vi "Create Indicator.vi"(0 "result cluster":refnum<vi>, 5 "vi reference":refnum<vi>, 7 "ctl refnum":refnum<vi>, 11 "error in":errorcluster) -> (15 "error out":errorcluster)   [LabVIEW 2021, in "Converter.lvlib"]
uses:
  Converter.lvlib
  <vilib>/Utility/miscctls.llb/LVPositionTypeDef.ctl
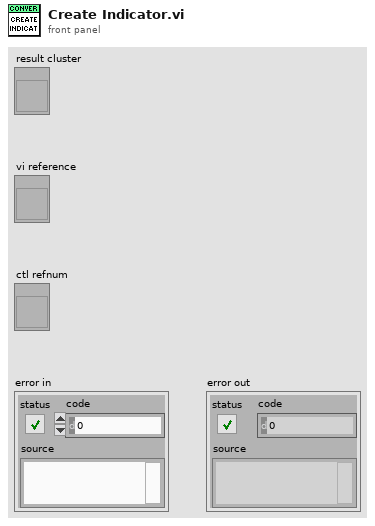
[diagram p1: front panel]
types:
  T1 = typedef "LVPositionTypeDef.ctl" = cluster{"Left":i32, "Top":i32}
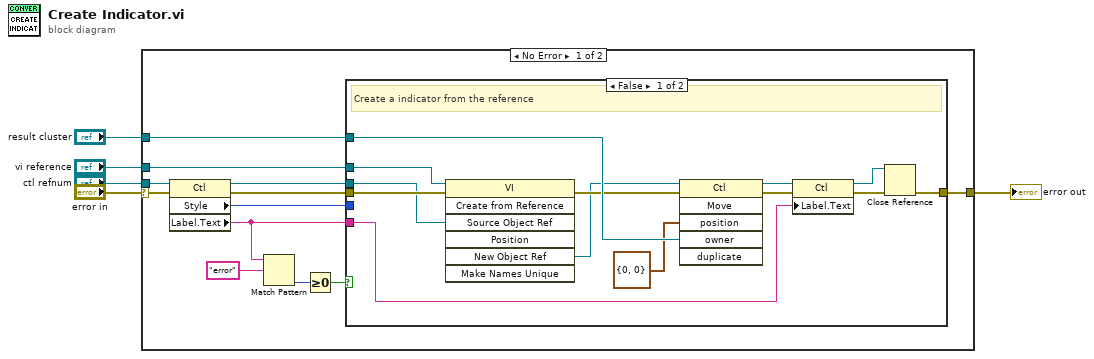
[diagram p0: block diagram]
diagram:
  n1 = case shown="No Error" "error in" {
    selector: "error in" -> [w17 w32]
    tunnel: "ctl refnum" -> [w16 _]
    tunnel: "vi reference" -> [w14 _]
    tunnel: [w10 w32] -> w2
    tunnel: "result cluster" -> [w8 _]
    frame No Error {
      n2 = property class="Ctl"(reference=w16, error in=w17) -> (reference out=w15:refnum<vi>, error out=w9:errorcluster, "Style"=w7:u32, "Label.Text"=w11:string)
      n3 = Match Pattern(string=w11, regular expression="error") -> (offset past match=w6:i32)  [unwired: 1 in, 3 out]
      n4 = Greater Or Equal To 0?(x=w6) -> (x >= 0?=w13:bool)
      n5 = case shown="False" w13 {
        tunnel: w7 -> [_ _]
        tunnel: w8 -> [w27 _]
        tunnel: w9 -> [w30 w31]
        tunnel: w15 -> [w26 _]
        tunnel: [w29 w31] -> w10
        tunnel: w11 -> [w28 _]
        tunnel: w14 -> [w25 _]
        frame False {
          # "Create a indicator from the reference"
          n6 = invoke class="VI" method="Create from Reference"(reference=w25, error in=w30, "Source Object Ref"=w26) -> (error out=w24:errorcluster, "New Object Ref"=w23:refnum<vi>)  [unwired: 4 in, 5 out]
          n7 = invoke class="Ctl" method="Move"(reference=w23, error in=w24, "position"=T1 {"Left"=0, "Top"=0}, "owner"=w27) -> (reference out=w19:refnum<vi>, error out=w21:errorcluster)  [unwired: 2 in, 4 out]
          n8 = property class="Ctl"(reference=w19, error in=w21, "Label.Text"=w28) -> (reference out=w18:refnum<vi>, error out=w20:errorcluster)
          n9 = Close Reference(reference=w18, error in (no error)=w20) -> (error out=w29:errorcluster)
        }
        frame True {
          # "Ignore it is error indicator"
        }
      }
    }
    frame Error {
    }
  }
  "error out" <- w2
